vi "8a.vi"() -> ()   [LabVIEW 2015]
panel:
  out "XY Graph 3":cluster{"Array":sgl[], "Array":sgl[]}(graph)
  out "XY Graph 2":cluster{"Array":sgl[], "Array":sgl[]}(graph)
  out "XY Graph":cluster{"Array":sgl[], "Array":sgl[]}(graph)
  in  "Cluster 2":cluster{"String":string, "Array":sgl[][]}
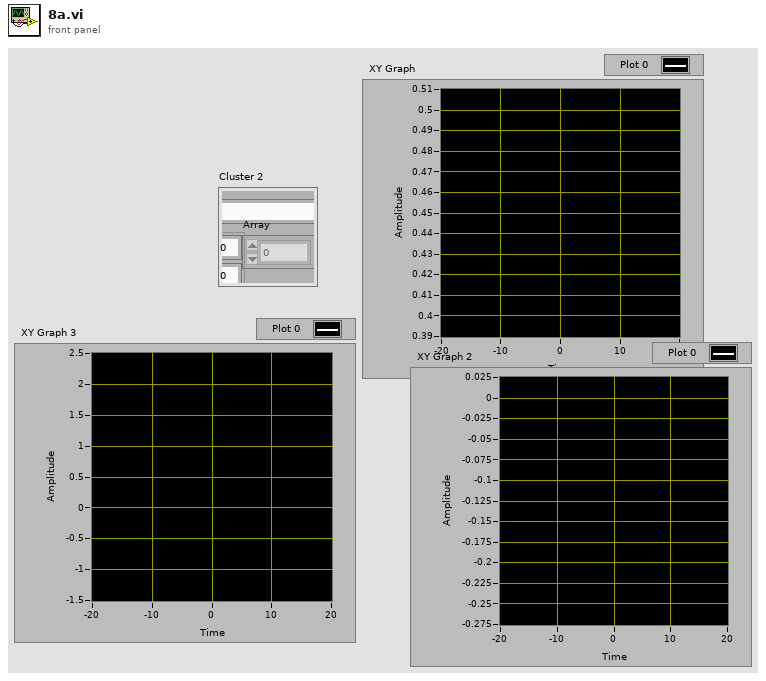
[diagram p1: front panel]
types:
  T1 = enum16{"open", "replace", "create", "open or create", "replace or create", "replace or create with confirmation"}
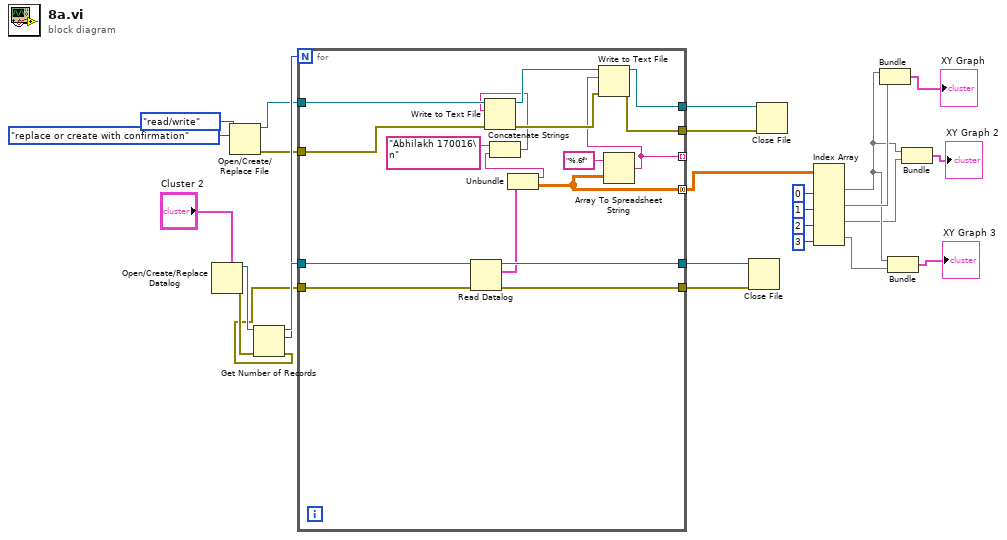
[diagram p0: block diagram]
diagram:
  n1 = Open/Create/Replace Datalog(5:"Cluster 2") -> (0:w22:errorcluster, 3:w23:refnum<k1>)  [unwired: 5 in, 1 out]
  n2 = Open/Create/Replace File(operation (0:open)=T1."replace or create with confirmation", access (0:read/write)=enum16{"read/write", "read-only", "write-only"}."read/write") -> (refnum out=w18:refnum<file>, error out=w17:errorcluster)  [unwired: 4 in, 1 out]
  n3 = Get Number of Records(4:w22, 7:w23) -> (0:w20:errorcluster, 2:w19:i64, 3:w21:refnum<k1>)
  n4 = for {
    N: w19 -> [_]
    tunnel: w20 -> [w41]
    tunnel: [w40] -> w24
    tunnel: w21 -> [w43]
    tunnel: [w42] -> w25
    tunnel: w18 -> [w38]
    tunnel: w17 -> [w37]
    tunnel: [w34] -> w16
    tunnel: [w33] -> w15
    tunnel: [w28] -> w12 mode=concatenating
    tunnel: [w27] -> _ mode=indexing
    n5 = Read Datalog(4:w41, 7:w43) -> (0:w40:errorcluster, 2:w39:cluster{"String":string, "Array":sgl[][]}, 3:w42:refnum<k1>)  [unwired: 1 in]
    n6 = Unbundle(w39) -> ("String"=w30:string, "Array"=w28:sgl[][])
    n7 = Concatenate Strings("Abhilakh 170016\n" ("string"), w30) -> (w29:string)
    n8 = Write to Text File(file (use dialog)=w38, text=w29, error in=w37) -> (refnum out=w36:refnum<file>, error out=w35:errorcluster)  [unwired: 1 in, 1 out]
    n9 = Array To Spreadsheet String(array=w28, 3:"%.6f" ("format string")) -> (spreadsheet string=w27:string)  [unwired: 1 in]
    n10 = Write to Text File(file (use dialog)=w36, text=w27, error in=w35) -> (refnum out=w34:refnum<file>, error out=w33:errorcluster)  [unwired: 1 in, 1 out]
  }
  n11 = Close File(refnum=w25, error in=w24) -> ()  [unwired: 2 out]
  n12 = Close File(refnum=w16, error in=w15) -> ()  [unwired: 2 out]
  n13 = Index Array(array=w12, index (col) #1=0 ("disabled index (col)"), index (col) #2=1 ("index (col)"), index (col) #3=2 ("index (col)"), index (col) #4=3 ("index (col)")) -> (element #1=w6:sgl[], element #2=w11:sgl[], element #3=w4:sgl[], element #4=w3:sgl[])  [unwired: 4 in]
  n14 = Bundle("Array"=w6, "Array"=w11) -> (→"XY Graph":cluster{"Array":sgl[], "Array":sgl[]})  [unwired: 1 in]
  n15 = Bundle("Array"=w6, "Array"=w3) -> (→"XY Graph 3":cluster{"Array":sgl[], "Array":sgl[]})  [unwired: 1 in]
  n16 = Bundle("Array"=w6, "Array"=w4) -> (→"XY Graph 2":cluster{"Array":sgl[], "Array":sgl[]})  [unwired: 1 in]
